vi "Get Now time.vi"() -> (2 "Time":string, 3 "Date":string)   [LabVIEW 2020]
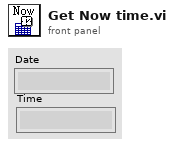
[diagram p1: front panel]
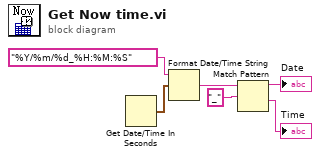
[diagram p0: block diagram]
diagram:
  n1 = Get Date/Time In Seconds() -> (seconds since 1Jan1904=w6:timestamp)
  n2 = Format Date/Time String(time format string (%c)="%Y/%m/%d_%H:%M:%S", seconds (now)=w6) -> (date/time string=w4:string)  [unwired: 1 in]
  n3 = Match Pattern(string=w4, regular expression="_") -> (before substring=→"Date":string, after substring=→"Time":string)  [unwired: 1 in, 2 out]
